vi "Read Session Attribute as String.vi"(8 "error in (no error)":errorcluster, 9 "Default Value (Empty)":string, 10 "Attribute Name":string, 11 "Session Handle in":refnum<data-value>) -> (0 "error out":errorcluster, 1 "Value":string, 2 "Exists":bool, 3 "Session Handle out":refnum<data-value>)   [LabVIEW 2020, in "G-Embedded-Python-Interpreter-Toolkit.lvlib"]
uses:
  G-Embedded-Python-Interpreter-Toolkit.lvlib
  bin/gepit.cp310.32.dll
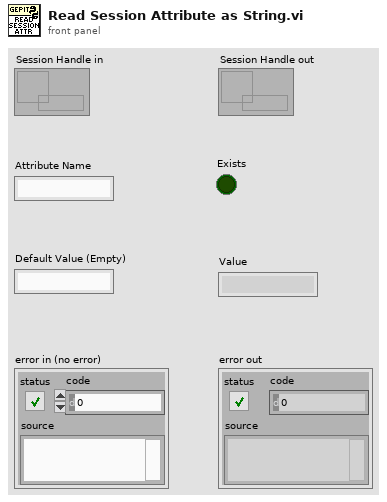
[diagram p1: front panel]
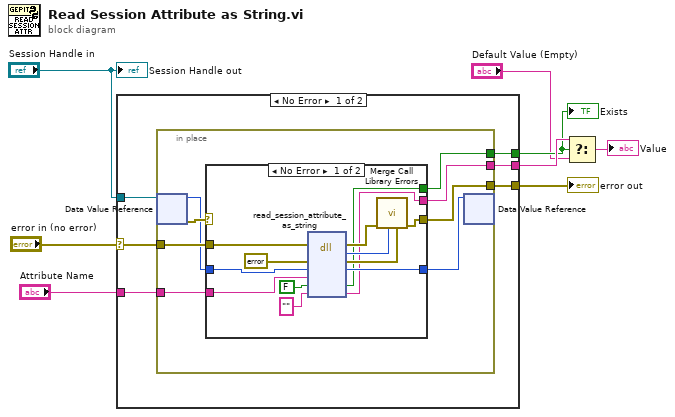
[diagram p0: block diagram]
diagram:
  n1 = case shown="No Error" "error in (no error)" {
    selector: "error in (no error)" -> [w13 w38]
    tunnel: "Session Handle in" -> [w14 _]
    tunnel: [w12 w38] -> w7
    tunnel: "Attribute Name" -> [w11 _]
    tunnel: [w10 _] -> w2
    tunnel: [w9 _] -> w4
    frame No Error {
      n2 = in-place {
        in-place-border: w13 -> [w21]
        in-place-border: [w18] -> w12
        in-place-border: w11 -> [w17]
        in-place-border: [w16] -> w10
        in-place-border: [w15] -> w9
        n3 = in-place-dvr #1(w14) -> (w20:u64, w22:errorcluster)
        n4 = case shown="No Error" w22 {
          selector: w22 -> [_ w36]
          tunnel: w21 -> [w31 _]
          tunnel: w20 -> [w30 w37]
          tunnel: [w29 w37] -> w19
          tunnel: [w28 w36] -> w18
          tunnel: w17 -> [w27 _]
          tunnel: [w25 _] -> w16
          tunnel: [w23 _] -> w15
          frame No Error {
            n5 = dll-call lib="C:/serenial/libraries/g-embedded-python-interpreter-toolkit/LabVIEW/bin/gepit.cp310.32.dll" fn="read_session_attribute_as_string"(error in=w31, "Error"=errorcluster {"status"=FALSE, "code"=0, "source"=""} ("error constant"), "Session"=w30, "Attribute Name"=w27, "Found"=FALSE, "Value"="") -> (error out=w34:errorcluster, "return type"=w33:i32, "Error"=w32:errorcluster, "Session"=w29:u64, "Found"=w25:bool, "Value"=w23:string)  [unwired: 3 in, 1 out]
            n6 = call "Merge Call Library Errors.vi"("Call Library Error"=w32, "Return Value"=w33, "error in"=w34) -> ("error out"=w28:errorcluster)  [unwired: 8 in]
          }
          frame Error {
          }
        }
        n7 = in-place-dvr #1(w19) -> ()  [unwired: 2 out]
      }
    }
    frame Error {
    }
  }
  "error out" <- w7
  "Exists" <- w2
  n8 = Select(t=w4, s=w2, f="Default Value (Empty)") -> (s? t:f=→"Value":string)
  "Session Handle out" <- "Session Handle in"
